vi "String Value.vi"(8 "error in":errorcluster, 9 "String In":string, 10 "Read/Write":enum16{"Write", "Read"}(ring), 11 "String in":refnum<vi>) -> (0 "error out":errorcluster, 1 "String Out":string)   [LabVIEW 2018]
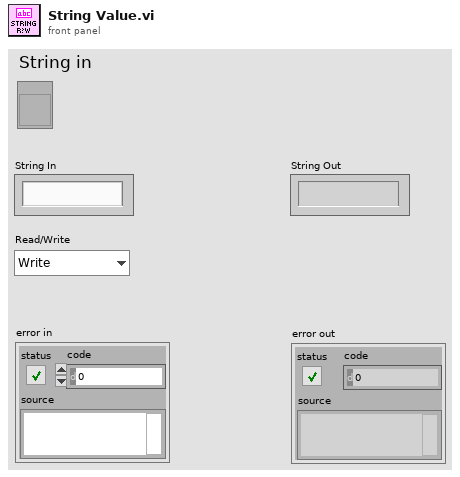
[diagram p1: front panel]
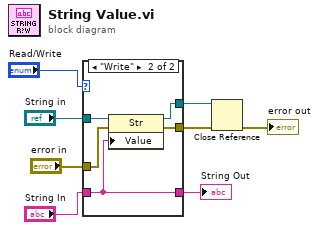
[diagram p0: block diagram]
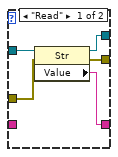
[diagram p2: hidden frame]
diagram:
  n1 = case shown="\"Write\"" "Read/Write" {
    tunnel: [w13 w18] -> w8
    tunnel: [w12 w17] -> w7
    tunnel: "String in" -> [w11 w16]
    tunnel: "error in" -> [w9 w15]
    tunnel: [w10 w14] -> w2
    tunnel: "String In" -> [_ w14]
    frame "Read" {
      n2 = property class="Str"(reference=w11, error in=w9) -> (reference out=w13:refnum<vi>, error out=w12:errorcluster, "Value"=w10:string)
    }
    frame "Write" {
      n3 = property class="Str"(reference=w16, error in=w15, "Value"=w14) -> (reference out=w18:refnum<vi>, error out=w17:errorcluster)
    }
  }
  "String Out" <- w2
  n4 = Close Reference(reference=w8, error in (no error)=w7) -> (error out=→"error out":errorcluster)
